vi "Start.vi"(8 "error in":errorcluster, 11 "Task Actor in":refnum<class "Task Actor.lvclass">) -> (0 "error out":errorcluster, 3 "Task Actor out":refnum<class "Task Actor.lvclass">)   [LabVIEW 2023, in "Task Actor.lvlib" / "Task Actor.lvclass"]
uses:
  Task Actor.lvclass
  Task Actor.lvclass/Task Actor.ctl
  <vilib>/ActorFramework/Actor/Actor.lvclass
  Measure and Stimulus Subsystems/Measure and Stimulus Subsystems.lvclass
  C:/Program Files/National Instruments/LabVIEW 2023/vi.lib/ActorFramework/Actor/Actor.lvclass
  D:/git/HAL/HAL GOOP4/Task/Task Actor/Task Actor/Task Actor.lvclass
  D:/git/HAL/HAL GOOP4/Task/ITask Actor/ITask Actor/ITask Actor.lvclass
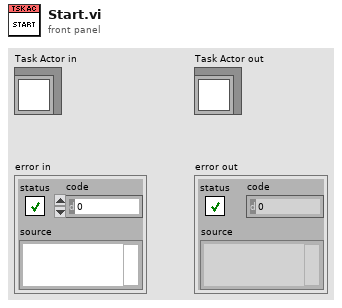
[diagram p1: front panel]
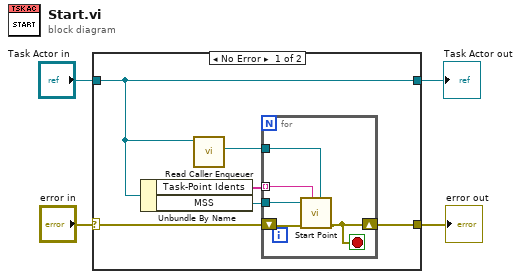
[diagram p0: block diagram]
diagram:
  n1 = case shown="No Error" "error in" {
    selector: "error in" -> [w6 w17]
    tunnel: "Task Actor in" -> [w10 w16]
    tunnel: [w5 w17] -> w3
    tunnel: [w10 w16] -> w1
    frame No Error {
      n2 = Unbundle By Name(w10) -> ("Task-Point Idents"=w9:string[], "MSS"=w8:refnum<class "Measure and Stimulus Subsystems.lvclass">)
      n3 = call <vilib>:"Read Caller Enqueuer.vi"("Actor"=w10) -> ("Caller Enqueuer"=w7:refnum<class "Message Enqueuer.lvclass">)  [unwired: 10 in]
      n4 = for {
        tunnel: w9 -> [w14] mode=indexing
        tunnel: w8 -> [w15]
        shift-right: [w12] -> w5
        shift-left: w6 -> [w13]
        tunnel: w7 -> [w11]
        stop <- w12 stop-if-true
        n5 = call "Start Point.vi"("Series Enqueuer"=w11, "Task-Point Ident"=w14, "error in"=w13, "MSS in"=w15) -> ("error out"=w12:errorcluster)  [unwired: 6 in, 1 out]
      }
    }
    frame Error {
    }
  }
  "error out" <- w3
  "Task Actor out" <- w1
